vi "DFS Sort Items.vi"(11 "Type Tree In":T1[](array[typedef])) -> (3 "DFS Sorted Type Tree":T1[](array[typedef]))   [LabVIEW 2018]
uses:
  <vilib>/Utility/Data Type/Type Definitions/Data Type.ctl
  <vilib>/Utility/Data Type/NI_Data Type.lvlib
  <resource>/Framework/Providers/LVClassByRef/Type Item.ctl
  <resource>/Framework/Providers/LVClassByRef/LVClassByRef.lvlib
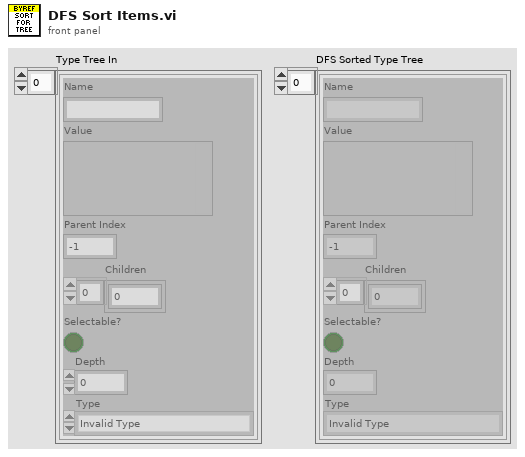
[diagram p1: front panel]
types:
  T1 = typedef "LVClassByRef.lvlib/Type Item.ctl" = cluster{"Name":string, "Value":variant, "Parent Index":i32, "Children":i32[], "Selectable?":bool, "Depth":i32, "Type":T2}
  T2 = typedef "NI_Data Type.lvlib/Data Type.ctl" = enum8{"Invalid Type", "Void", "I8", "I16", "I32", "I64", "U8", "U16", "U32", "U64", "Single Float", "Double Float", "Extended Float", "Single Complex", "Double Complex", "Extended Complex", "Enum U8", "Enum U16", "Enum U32", "Enum U64", "Single Float With Unit", "Double Float With Unit", "Extended Float With Unit", "Single Complex with Unit", "Double Complex with Unit", "Extended Complex with Unit", "Boolean", "String", "Path", "Picture", "Tag", "Array", "Cluster", "Variant", "LV Variant", "Waveform", "Timestamp", "Digital Waveform", "Digital Data", "ExpressData", "Refnum", "External Data", "VI", "Poly VI", "LabVIEW Class Instance", "Fixed Point"}
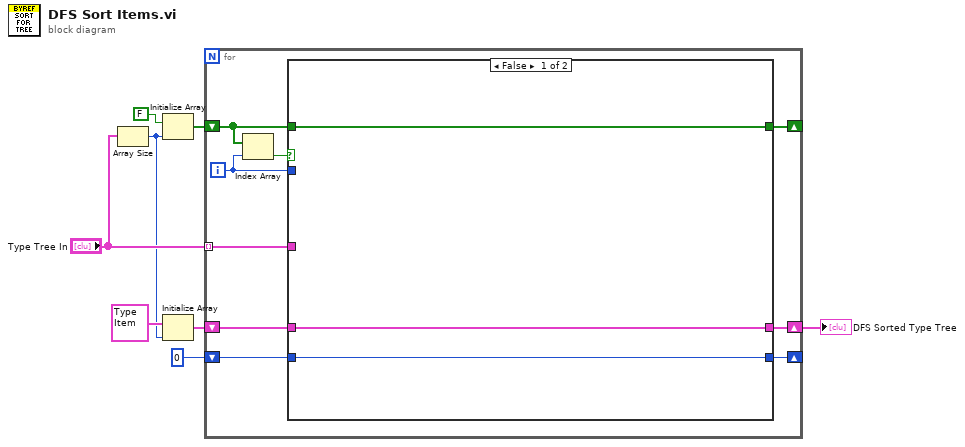
[diagram p0: block diagram]
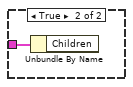
[diagram p2: hidden frame]
diagram:
  n1 = Array Size(array="Type Tree In") -> (size(s)=w4:i32)
  n2 = Initialize Array(FALSE, w4) -> (w7:bool[])
  n3 = Initialize Array(T1 {"Name"="", "Value"=variant, "Parent Index"=-1, "Children"=[], "Selectable?"=FALSE, "Depth"=0, "Type"=enum."Invalid Type"} ("Type Item"), w4) -> (w3:T1[])
  n4 = for {
    tunnel: "Type Tree In" -> [w11] mode=indexing
    shift-right: [w13] -> w1
    shift-left: w3 -> [w14]
    shift-right: [w15] -> _
    shift-left: w7 -> [w16]
    shift-right: [w9] -> _
    shift-left: 0 -> [w10]
    i -> [w12]
    n5 = Index Array(array=w16, index=w12) -> (element=w17:bool)
    n6 = case shown="False" w17 {
      tunnel: w16 -> [w20 _]
      tunnel: [w20 _] -> w15
      tunnel: w14 -> [w19 _]
      tunnel: [w19 _] -> w13
      tunnel: w12 -> [_ _]
      tunnel: w11 -> [_ w21]
      tunnel: w10 -> [w18 _]
      tunnel: [w18 _] -> w9
      frame False {
      }
      frame True {
        n7 = Unbundle By Name(w21) -> ()  [unwired: 1 out]
      }
    }
  }
  "DFS Sorted Type Tree" <- w1
